vi "System.vi"(8 "error in (no error)":errorcluster, 11 "VolatusConfig in":refnum<class "VolatusConfig.lvclass">) -> (0 "error out":errorcluster, 2 "System":refnum<class "System Config.lvclass">, 3 "VolatusConfig out":refnum<class "VolatusConfig.lvclass">)   [LabVIEW 2020, in "VolatusConfig.lvlib" / "VolatusConfig.lvclass"]
uses:
  VolatusConfig.lvclass
  VolatusConfig.lvclass/VolatusConfig.ctl
  Meta Type.ctl
  VolatusConfig.lvlib
  System/System Config.lvclass
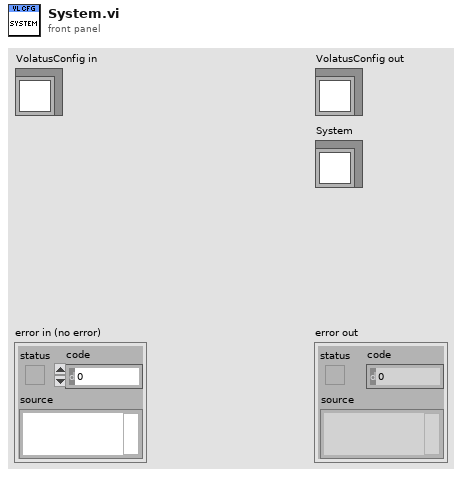
[diagram p1: front panel]
types:
  T1 = typedef "VolatusConfig.lvlib/Meta Type.ctl" = enum16{"UNKNOWN", "VL_System", "VL_Cluster", "VL_Node", "VL_Task", "VL_Group", "VL_Channel", "VL_Task_List", "VL_Scaling", "VL_Sensor", "VL_Sensor_List", "VL_Scale"}
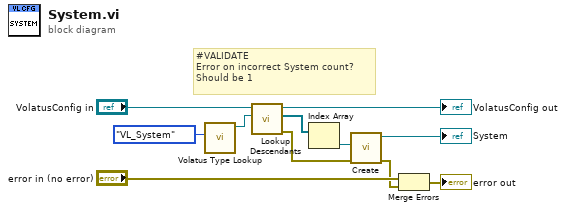
[diagram p0: block diagram]
diagram:
  # "#VALIDATE\nError on incorrect System count?\nShould be 1"
  n1 = call "Volatus Type Lookup.vi"("Meta Type"=Meta_Type."VL_System") -> ("Config Lookup out"=w7:refnum<class "Config Lookup.lvclass">)  [unwired: 9 in, 1 out]
  n2 = call "Lookup Descendants.vi"("Lookup"=w7, "VolatusConfig in"="VolatusConfig in") -> ("error out"=w8:errorcluster, "Descendants"=w6:refnum<class "Config Element.lvclass">[], "VolatusConfig out"=→"VolatusConfig out":refnum<class "VolatusConfig.lvclass">)  [unwired: 7 in]
  n3 = Index Array(array=w6) -> (element=w9:refnum<class "Config Element.lvclass">)  [unwired: 1 in]
  n4 = call "Create.vi"("error in (no error)"=w8, "Element"=w9) -> ("error out"=w1:errorcluster, "System out"=→"System":refnum<class "System Config.lvclass">)  [unwired: 8 in]
  n5 = Merge Errors("error in (no error)", w1) -> (→"error out":errorcluster)
